vi "Panel Helper.vi"(8 "Error In":errorcluster) -> (0 "Error Out":errorcluster, 2 "Panel Events":T1, 3 "Panel Helper out":refnum<class "Panel Helper.lvclass">)   [LabVIEW 2023, in "Panel Actor.lvlib" / "Panel.lvlib" / "Panel Helper.lvclass"]
doc: "Instantiates the Panel Helper.\n\n<B>Error In:</B> Describes error conditions that occur before this node runs.\n\n<B>Panel Helper Out:</B> New Panel Helper object.\n<B>Panel Events:</B> Associated panel events.\n<B>Error Out:</B> Contains error information.\n----\nPlease see the following web address for additional documentation and tutorial information:\nhttp://www.mooregoodideas.com/mgi-panel-manager/\n\nAuthor: Derek Trepanier\n\nCopyright (c) 2018, Moore Good Ideas, Inc.\n\nAll rights reserved.\n\nRedistribution and use in source and binary forms, with or without modification, are permitted provided that the following conditions are met:\n\n * Redistributions of source code must retain the above copyright notice, this list of conditions and the following disclaimer.\n * Redistributions in binary form must reproduce the above copyright notice, this list of conditions and the following disclaimer in the documentation and/or other materials provided with the distribution.\n * Neither the name of Moore Good Ideas, Inc. nor the names of its contributors may be used to endorse or promote products derived from this software without specific prior written permission.\n\nTHIS SOFTWARE IS PROVIDED BY THE COPYRIGHT HOLDERS AND CONTRIBUTORS \"AS IS\" AND ANY EXPRESS OR IMPLIED WARRANTIES, INCLUDING, BUT NOT LIMITED TO, THE IMPLIED WARRANTIES OF MERCHANTABILITY AND FITNESS FOR A PARTICULAR PURPOSE ARE DISCLAIMED. IN NO EVENT SHALL THE COPYRIGHT OWNER OR CONTRIBUTORS BE LIABLE FOR ANY DIRECT, INDIRECT, INCIDENTAL, SPECIAL, EXEMPLARY, OR CONSEQUENTIAL DAMAGES (INCLUDING, BUT NOT LIMITED TO, PROCUREMENT OF SUBSTITUTE GOODS OR SERVICES; LOSS OF USE, DATA, OR PROFITS; OR BUSINESS INTERRUPTION) HOWEVER CAUSED AND ON ANY THEORY OF LIABILITY, WHETHER IN CONTRACT, STRICT LIABILITY, OR TORT (INCLUDING NEGLIGENCE OR OTHERWISE) ARISING IN ANY WAY OUT OF THE USE OF THIS SOFTWARE, EVEN IF ADVISED OF THE POSSIBILITY OF SUCH DAMAGE."
uses:
  Panel Helper.lvclass
  Panel Events.ctl
  Events.ctl
  Panel Updater/Panel Updater.lvclass
  Panel Helper.lvclass/Panel Helper.ctl
  Deferer/Deferer.lvclass
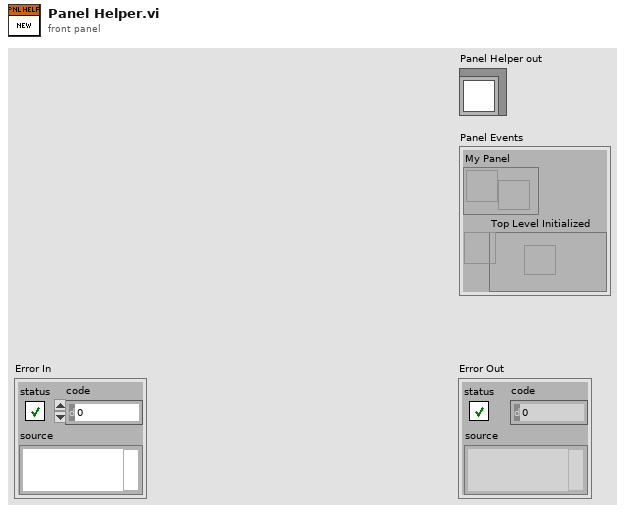
[diagram p1: front panel]
types:
  T1 = typedef "Panel Actor.lvlib/Panel.lvlib/Panel Helper.lvclass/Panel Events.ctl" = cluster{"My Panel":refnum<user-event>, "Top Level Initialized":refnum<user-event>}
  T2 = typedef "Panel Actor.lvlib/Panel.lvlib/Panel Helper.lvclass/Events.ctl" = enum16{"Initialized", "Shown", "Hidden", "Closed"}
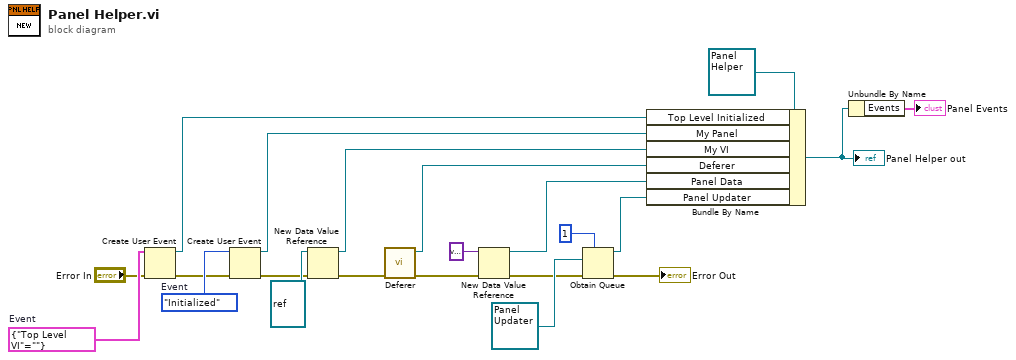
[diagram p0: block diagram]
diagram:
  w6 = cluster{"Top Level VI":string} {"Top Level VI"=""}  # Event
  w11 = Events."Initialized"  # Event
  n1 = Create User Event(user event datatype=w6, error in="Error In") -> (user event=w1:refnum<user-event>, error out=w2:errorcluster)
  n2 = Create User Event(user event datatype=w11, error in=w2) -> (user event=w10:refnum<user-event>, error out=w19:errorcluster)
  n3 = New Data Value Reference(data value=refnum<vi> refnum ("VI Refnum"), error in=w19) -> (data value reference=w21:refnum<data-value>, error out=w9:errorcluster)
  n4 = call "Deferer.vi"("error in (no error)"=w9) -> ("error out"=w8:errorcluster, "Deferer out"=w7:refnum<class "Deferer.lvclass">)  [unwired: 9 in]
  n5 = New Data Value Reference(data value=variant, error in=w8) -> (data value reference=w17:refnum<data-value>, error out=w13:errorcluster)
  n6 = Obtain Queue(max queue size (-1, unlimited)=1, element data type=refnum<class "Panel Updater.lvclass"> refnum ("Panel.lvlib:Panel Updater.lvclass"), error in (no error)=w13) -> (queue out=w14:refnum<queue>, error out=→"Error Out":errorcluster)  [unwired: 2 in, 1 out]
  n7 = Bundle By Name(cluster=refnum<class "Panel Helper.lvclass"> refnum ("Helper in"), "Top Level Initialized"=w1, "My Panel"=w10, "My VI"=w21, "Deferer"=w7, "Panel Data"=w17, "Panel Updater"=w14) -> (w5:refnum<class "Panel Helper.lvclass">)
  "Panel Helper out" <- w5
  n8 = Unbundle By Name(w5) -> ("Events"=→"Panel Events":T1)
